vi "AB_API Get Project Item Reference.vi"(6 "Exclude dependencies":bool=TRUE, 7 "TargetItem Refnum":refnum<vi>, 8 "error in (no error)":errorcluster, 9 "Type":string, 10 "Name":string, 11 "Project Refnum":refnum<vi>) -> (0 "error out":errorcluster, 2 "found?":bool, 3 "ProjectItem Refnum":refnum<vi>)   [LabVIEW 2020]
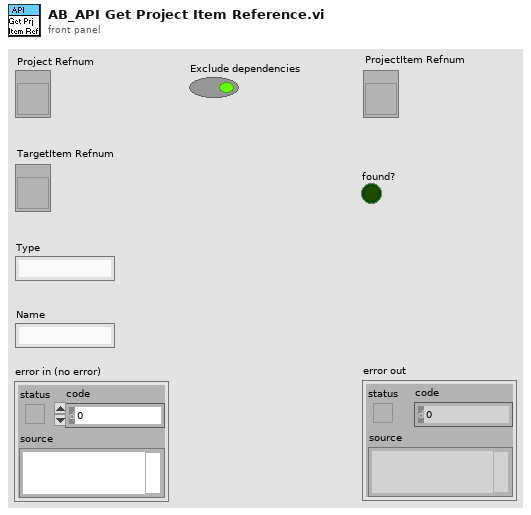
[diagram p1: front panel]
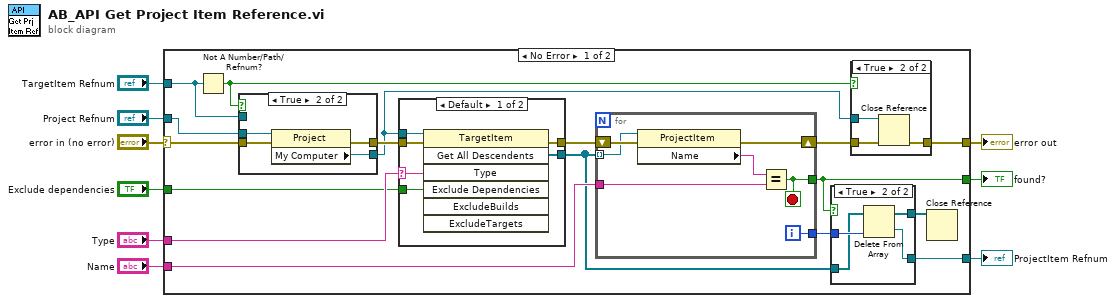
[diagram p0: block diagram]
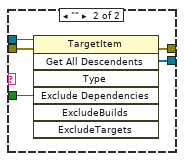
[diagram p4: hidden frame]
diagram:
  n1 = case shown="No Error" "error in (no error)" {
    selector: "error in (no error)" -> [w22 w60]
    tunnel: "Project Refnum" -> [w26 _]
    tunnel: "TargetItem Refnum" -> [w25 _]
    tunnel: [w17 w60] -> w7
    tunnel: [w13 _] -> w6
    tunnel: "Name" -> [w21 _]
    tunnel: "Type" -> [w20 _]
    tunnel: "Exclude dependencies" -> [w19 _]
    tunnel: [w12 _] -> w1
    frame No Error {
      n2 = Not A Number/Path/Refnum?(number/path/refnum=w25) -> (NaN/Path/Refnum?=w11:bool)
      n3 = case shown="True" w11 {
        tunnel: [w55 w59] -> w10
        tunnel: [w54 w58] -> w23
        tunnel: w26 -> [_ w57]
        tunnel: w25 -> [w55 _]
        tunnel: w22 -> [w54 w56]
        frame False {
        }
        frame True {
          n4 = property class="Project"(reference=w57, error in=w56) -> (error out=w58:errorcluster, "My Computer"=w59:refnum<vi>)  [unwired: 1 out]
        }
      }
      n5 = case shown="Default" w20 {
        selector: w20 -> [w36 _]
        tunnel: [w41 w46] -> w24
        tunnel: w19 -> [w40 w45]
        tunnel: w10 -> [w39 w44]
        tunnel: [w38 w43] -> w14
        tunnel: w23 -> [w37 w42]
        frame Default {
          n6 = invoke class="TargetItem" method="Get All Descendents"(reference=w39, error in=w37, "Type"=w36, "Exclude Dependencies"=w40) -> (error out=w41:errorcluster, "All Descendents"=w38:refnum<vi>[])  [unwired: 3 in, 5 out]
        }
        frame "" {
          n7 = invoke class="TargetItem" method="Get All Descendents"(reference=w44, error in=w42, "Exclude Dependencies"=w45) -> (error out=w46:errorcluster, "All Descendents"=w43:refnum<vi>[])  [unwired: 4 in, 5 out]
        }
      }
      n8 = for {
        tunnel: w14 -> [w52] mode=indexing
        shift-right: [w51] -> w18
        shift-left: w24 -> [w53]
        tunnel: w21 -> [w49]
        tunnel: [w48] -> w13
        tunnel: [w47] -> w15
        i -> [w47]
        stop <- w48 stop-if-true
        n9 = property class="ProjectItem"(reference=w52, error in=w53) -> (error out=w51:errorcluster, "Name"=w50:string)  [unwired: 1 out]
        n10 = Equal?(x=w50, y=w49) -> (x = y?=w48:bool)
      }
      n11 = case shown="True" w13 {
        tunnel: w15 -> [_ w31]
        tunnel: w14 -> [w27 w30]
        tunnel: [w27 w29] -> w16
        tunnel: [_ w28] -> w12
        frame False {
        }
        frame True {
          n12 = Delete From Array(array=w30, index=w31) -> (deleted portion=w28:refnum<vi>, array with subset deleted=w29:refnum<vi>[])  [unwired: 1 in]
        }
      }
      n13 = case shown="True" w11 {
        tunnel: w18 -> [w32 w35]
        tunnel: w10 -> [_ w33]
        tunnel: [w32 w34] -> w17
        frame False {
        }
        frame True {
          n14 = Close Reference(reference=w33, error in (no error)=w35) -> (error out=w34:errorcluster)
        }
      }
      n15 = Close Reference(reference=w16) -> ()  [unwired: 1 in, 1 out]
    }
    frame Error {
    }
  }
  "ProjectItem Refnum" <- w1
  "error out" <- w7
  "found?" <- w6
